vi "WebCam.InitPreview.vi"(0 "Handle":i32, 11 "ErrorIn":errorcluster) -> (4 "HandleOut":i32, 15 "ErrorOut":errorcluster)   [LabVIEW 2021]
uses:
  User32.WebCam_WM_Events.ctl
  User32.SendMessageA_num.vi
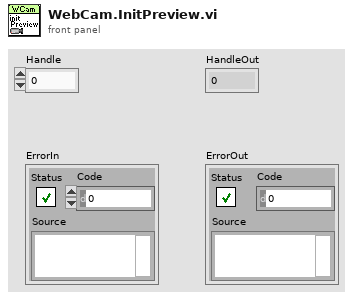
[diagram p1: front panel]
types:
  T1 = typedef "User32.WebCam_WM_Events.ctl" = i32
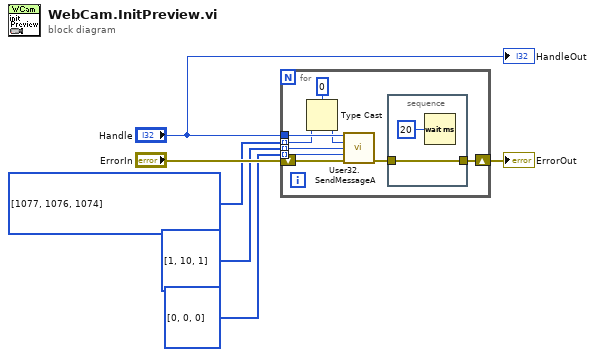
[diagram p0: block diagram]
diagram:
  w4 = T1[] [1077, 1076, 1074] items=["WM_CAP_DRIVER_CONNECT"=1034, "WM_CAP_DRIVER_DISCONNECT"=1035, "WM_CAP_EDIT_COPY"=1054, "WM_CAP_SEQUENCE"=1086, "WM_CAP_FILE_SAVEAS"=1047, "WM_CAP_SET_SCALE"=1077, "WM_CAP_SET_PREVIEWRATE"=1076, "WM_CAP_SET_PREVIEW"=1074, "WM_CAP_SET_OVERLAY"=1075, "WM_CAP_FILE_SAVEDIB"=1049]
  n1 = for {
    shift-right: [w13] -> w5
    shift-left: "ErrorIn" -> [w15]
    tunnel: "Handle" -> [w12]
    tunnel: w4 -> [w9] mode=indexing
    tunnel: i32[] [1, 10, 1] -> [w11] mode=indexing
    tunnel: i32[] [0, 0, 0] -> [w10] mode=indexing
    n2 = Type Cast(type=0, x=w9) -> (*(type *) &x=w7:i32)
    n3 = call-poly "User32.SendMessageA.vi"("HWnd"=w12, "Msg"=w7, "WParam"=w11, "LParam"=w10, "ErrorIn"=w15) -> ("ErrorOut"=w14:errorcluster)  [unwired: 9 in, 1 out]
    n4 = stacked-sequence {
      tunnel: w14 -> [w17]
      tunnel: [w17] -> w13
      frame #0 {
        n5 = Wait (ms)(milliseconds to wait=u32 20) -> ()  [unwired: 1 out]
      }
    }
  }
  "ErrorOut" <- w5
  "HandleOut" <- "Handle"
